vi "题目8.vi"() -> ()   [LabVIEW 2017]
panel:
  out "Y":dbl
  in  "N":dbl
  in  "M":dbl
  in  "X":dbl
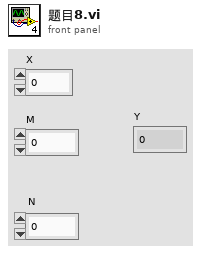
[diagram p1: front panel]
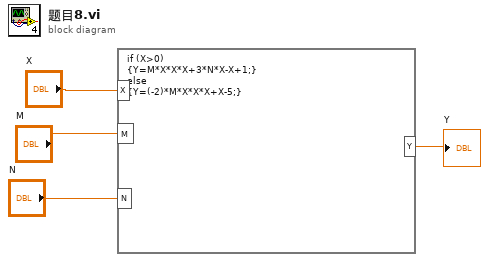
[diagram p0: block diagram]
diagram:
  n1 = formula code="if (X>0)\n{Y=M*X*X*X+3*N*X-X+1;}\nelse\n{Y=(-2)*M*X*X*X+X-5;}"("X"="X", "M"="M", "N"="N") -> ("Y"=→"Y":dbl)
